vi "Test1.vi"   [LabVIEW 2014, in "Queue_Library.lvlib"]
uses:
  Queue_Library.lvlib
  Enqueue_Queue_Single.vi
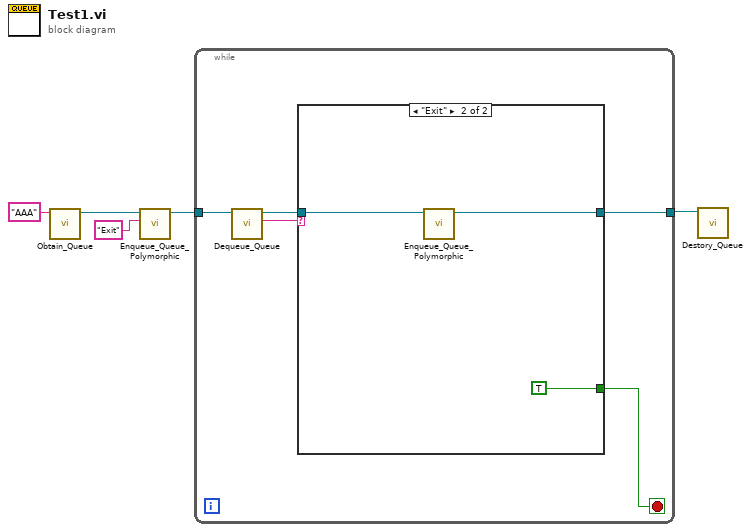
[diagram p0: block diagram]
diagram:
  n1 = call "Obtain_Queue.vi"("Name"="AAA") -> ("queue out"=w4:refnum<queue>)  [unwired: 9 in, 1 out]
  n2 = call-poly "Enqueue_Queue_Polymorphic.vi"("Command"="Exit", "queue In"=w4) -> ("queue Out"=w3:refnum<queue>)  [unwired: 8 in, 1 out]
  n3 = while {
    tunnel: w3 -> [w9]
    tunnel: [w10] -> w5
    stop <- w6 stop-if-true
    n4 = call "Dequeue_Queue.vi"("queue In"=w9) -> ("Command"=w7:string, "queue Out"=w8:refnum<queue>)  [unwired: 7 in, 2 out]
    n5 = case shown="\"Exit\"" w7 {
      tunnel: w8 -> [w11 w14]
      tunnel: [w11 w13] -> w10
      tunnel: [_ TRUE] -> w6
      frame Default {
      }
      frame "Exit" {
        n6 = call-poly "Enqueue_Queue_Polymorphic.vi"("queue In"=w14) -> ("queue Out"=w13:refnum<queue>)  [unwired: 9 in, 1 out]
      }
    }
  }
  n7 = call "Destory_Queue.vi"("queue In"=w5) -> ()  [unwired: 10 in, 1 out]
